vi "ChangeLatency.vi"() -> ()   [LabVIEW 2017]
uses:
  <vilib>/registry/registry.llb/Registry RtKey.ctl
  <vilib>/registry/registry.llb/Read Registry Value Simple STR.vi
  <vilib>/registry/registry.llb/Write Registry Value Simple STR.vi
panel:
  out "simple data type":enum16{"String", "Binary", "DWORD"}(ring)
  out "String/Binary data":string
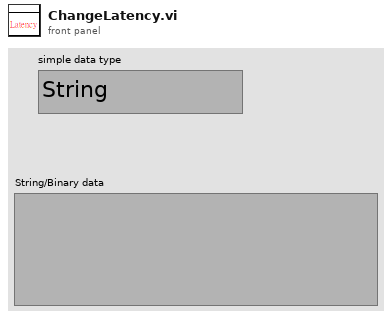
[diagram p1: front panel]
types:
  T1 = typedef "Registry RtKey.ctl" = enum32{"HKEY_CLASSES_ROOT", "HKEY_CURRENT_USER", "HKEY_LOCAL_MACHINE", "HKEY_USERS", "HKEY_PERFORMANCE_DATA", "HKEY_CURRENT_CONFIG", "HKEY_DYN_DATA"}
  T2 = typedef "Registry refnum.ctl" = refnum<k1>
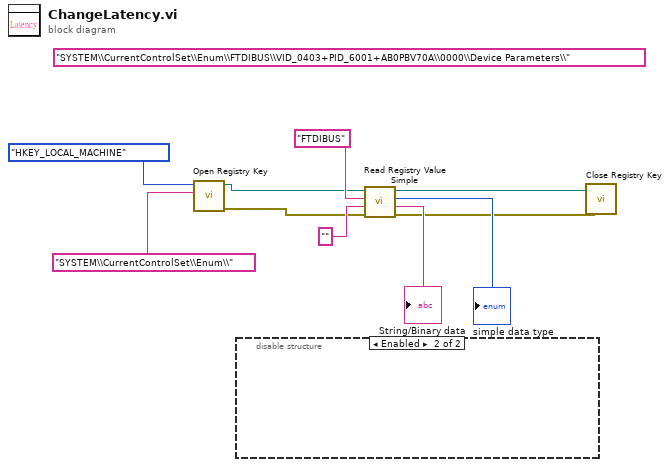
[diagram p0: block diagram]
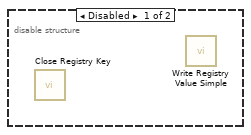
[diagram p2: hidden frame]
diagram:
  (unwired) "SYSTEM\\CurrentControlSet\\Enum\\FTDIBUS\\VID_0403+PID_6001+AB0PBV70A\\0000\\Device Parameters\\" ("subkey")
  n1 = call <vilib>:"Open Registry Key.vi"("subkey"="SYSTEM\\CurrentControlSet\\Enum\\", "root key (HKEY_LOCAL_MACHINE)"=Registry_RtKey."HKEY_LOCAL_MACHINE") -> ("error out"=w5:errorcluster, "refnum out"=w6:T2)  [unwired: 8 in]
  n2 = disable-structure shown="Enabled" {
    frame Disabled {
      n3 = call <vilib>:"Close Registry Key.vi"() -> ()  [unwired: 7 in, 1 out]
      n4 = call-poly <vilib>:"Write Registry Value Simple.vi"() -> ()  [unwired: 8 in, 2 out]
    }
    frame Enabled {
    }
  }
  n5 = call-poly <vilib>:"Read Registry Value Simple.vi"("error in (no error)"=w5, "default data"="", "value"="FTDIBUS", "refnum"=w6) -> ("error out"=w1:errorcluster, "String/Binary data"=→"String/Binary data":string, "simple data type"=→"simple data type":enum16{"String", "Binary", "DWORD"}, "refnum out"=w2:T2)  [unwired: 2 in]
  n6 = call <vilib>:"Close Registry Key.vi"("error in (no error)"=w1, "refnum"=w2) -> ()  [unwired: 5 in, 1 out]
